vi "Parse Label.vi"(0 "Stage Controller StepMotor in":refnum<class "Stage Controller StepMotor.lvclass">, 5 "Label.Text":string, 11 "error in (no error)":errorcluster) -> (4 "Stage Controller StepMotor out":refnum<class "Stage Controller StepMotor.lvclass">, 6 "Stage Label":string, 8 "Increase?":bool=TRUE, 10 "Big Step?":bool, 15 "error out":errorcluster)   [LabVIEW 2020, in "Stage.lvlib" / "Stage Controller StepMotor.lvlib" / "Stage Controller StepMotor.lvclass"]
uses:
  Stage Controller StepMotor.lvclass
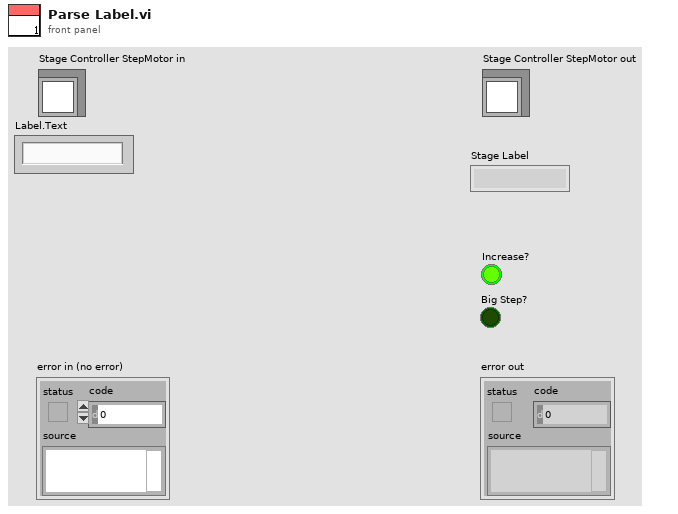
[diagram p1: front panel]
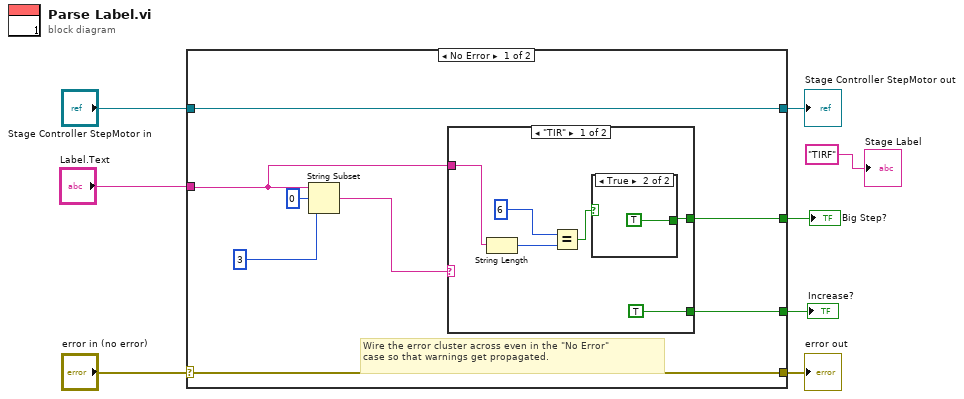
[diagram p0: block diagram]
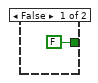
[diagram p2: hidden frame]
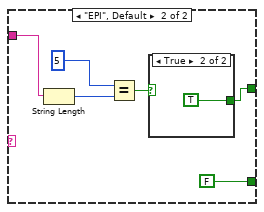
[diagram p3: hidden frame]
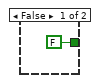
[diagram p4: hidden frame]
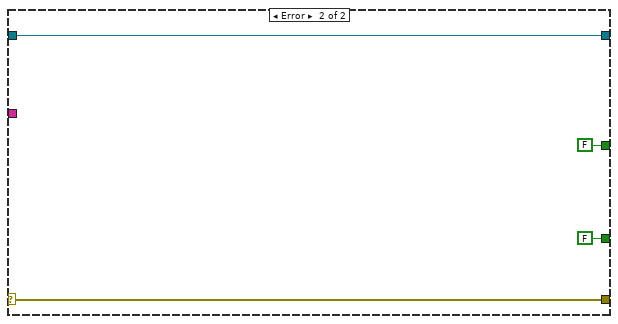
[diagram p5: hidden frame]
diagram:
  n1 = case shown="No Error" "error in (no error)" {
    selector: "error in (no error)" -> [w15 w36]
    tunnel: [w15 w36] -> w7
    tunnel: [w16 w35] -> w5
    tunnel: "Stage Controller StepMotor in" -> [w16 w35]
    tunnel: "Label.Text" -> [w10 _]
    tunnel: [w12 FALSE ("Increase?")] -> w3
    tunnel: [w9 FALSE ("Increase?")] -> w2
    frame No Error {
      # "Wire the error cluster across even in the \"No Error\"\ncase so that warnings get propagated."
      n2 = String Subset(string=w10, offset (0)=0, length (rest)=3 ("length (rest)")) -> (substring=w11:string)
      n3 = case shown="\"TIR\"" w11 {
        tunnel: [TRUE ("Increase?") FALSE ("Increase?")] -> w12
        tunnel: w10 -> [w18 w27]
        tunnel: [w17 w25] -> w9
        frame "TIR" {
          n4 = String Length(string=w18) -> (length=w21:i32)
          n5 = Equal?(x=6, y=w21) -> (x = y?=w19:bool)
          n6 = case shown="True" w19 {
            tunnel: [FALSE ("Increase?") TRUE ("Increase?")] -> w17
            frame False {
            }
            frame True {
            }
          }
        }
        frame "EPI", Default {
          n7 = String Length(string=w27) -> (length=w29:i32)
          n8 = Equal?(x=5, y=w29) -> (x = y?=w26:bool)
          n9 = case shown="True" w26 {
            tunnel: [FALSE ("Increase?") TRUE ("Increase?")] -> w25
            frame False {
            }
            frame True {
            }
          }
        }
      }
    }
    frame Error {
    }
  }
  "error out" <- w7
  "Stage Controller StepMotor out" <- w5
  "Increase?" <- w3
  "Big Step?" <- w2
  "Stage Label" <- "TIRF" ("Stage Label")
